vi "Destroy.vi"(8 "Error In":errorcluster) -> (0 "Error Out":errorcluster)   [LabVIEW 2018, in "TracerLibrary.lvlib" / "Tracer.lvclass"]
uses:
  Tracer.lvclass
  protected/Tracer_ClassAttributes.vi
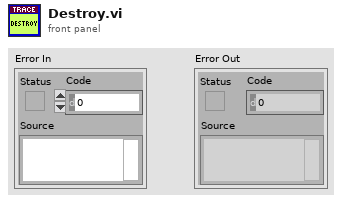
[diagram p1: front panel]
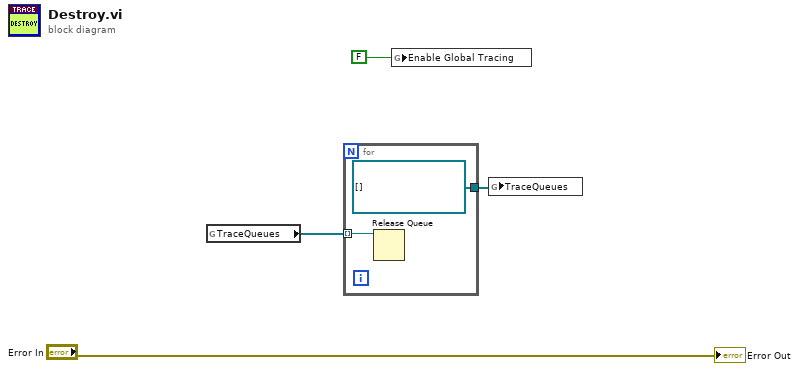
[diagram p0: block diagram]
diagram:
  n1 = global read "Tracer_ClassAttributes.vi" "TraceQueues"() -> (w2:refnum<queue>[])
  n2 = for {
    tunnel: w2 -> [w6] mode=indexing
    tunnel: [refnum<queue>[] [] ("TraceQueues")] -> w3
    n3 = Release Queue(queue=w6) -> ()  [unwired: 2 in, 3 out]
  }
  n4 = global write "Tracer_ClassAttributes.vi" "Enable Global Tracing"(FALSE ("TRACE Enable")) -> ()
  n5 = global write "Tracer_ClassAttributes.vi" "TraceQueues"(w3) -> ()
  "Error Out" <- "Error In"
